vi "Turn to angle.vi"(8 "Start Time":u32, 9 "Range of accuracy":sgl, 10 "desired angle":sgl) -> (1 "In Range?":bool, 2 "coerced(x)":dbl)   [LabVIEW 2020]
doc: "turn to angle calculation in degrees"
uses:
  Robot Global Data.vi
panel:
  out "Degrees per second":dbl
  out "Diffrence":dbl
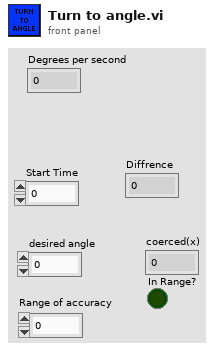
[diagram p1: front panel]
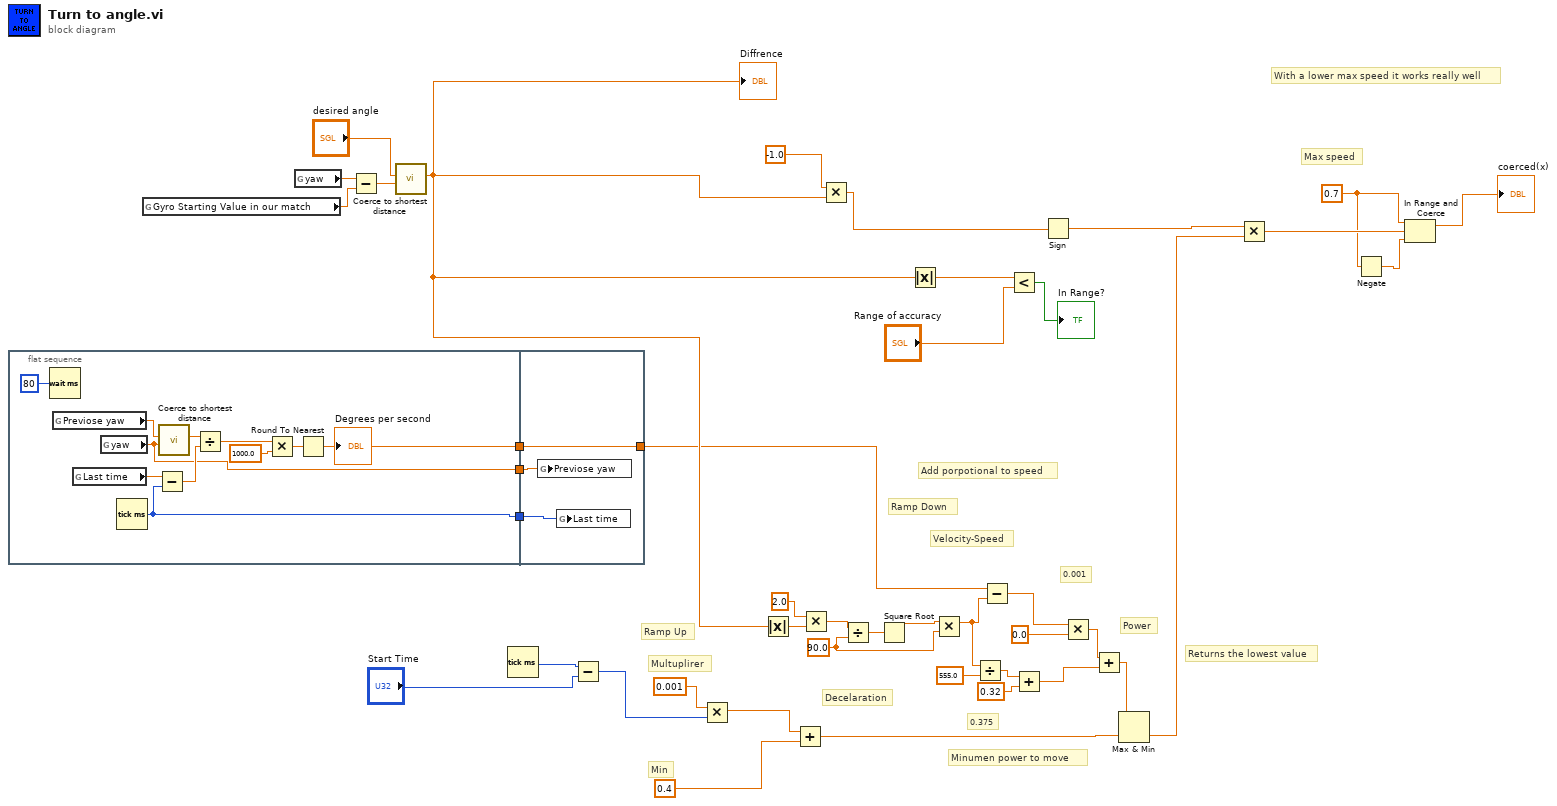
[diagram p0: block diagram]
diagram:
  w16 = 90.0 ("x")
  w33 = 0.7 ("t")
  # "0.375"
  # "0.001"
  # "Power"
  # "Minumen power to move"
  # "Add porpotional to speed"
  # "Ramp Down"
  # "Velocity-Speed"
  # "Decelaration"
  # "With a lower max speed it works really well"
  # "Multuplirer"
  # "Min"
  # "Ramp Up"
  # "Returns the lowest value"
  # "Max speed"
  n1 = flat-sequence {
    tunnel: [w51] -> w23
    tunnel: [w45] -> w22
    tunnel: [w43] -> w10
    tunnel: w23 -> [w56]
    tunnel: w22 -> [w55]
    tunnel: [w54] -> w11
    tunnel: w10 -> [w54]
    frame #0 {
      n2 = Wait (ms)(milliseconds to wait=u32 80) -> ()  [unwired: 1 out]
      n3 = global read "Robot Global Data.vi" "Previose yaw"() -> (w46:dbl)
      n4 = global read "Robot Global Data.vi" "Last time"() -> (w53:dbl)
      n5 = global read "Robot Global Data.vi" "yaw"() -> (w45:dbl)
      n6 = Tick Count (ms)() -> (millisecond timer value=w51:u32)
      n7 = Subtract(x=w53, y=w51) -> (x-y=w52:dbl)
      n8 = call "Coerce to shortest distance.vi"("Angle 2"=w45, "Angle 1"=w46) -> ("Shortest distance"=w44:dbl)  [unwired: 9 in]
      n9 = Divide(x=w44, y=w52) -> (x/y=w50:dbl)
      n10 = Multiply(x=w50, y=1000.0) -> (x*y=w47:dbl)
      n11 = Round To Nearest(number=w47) -> (nearest integer value=w43:dbl)
      "Degrees per second" <- w43
    }
    frame #1 {
      n12 = global write "Robot Global Data.vi" "Previose yaw"(w55) -> ()
      n13 = global write "Robot Global Data.vi" "Last time"(w56) -> ()
    }
  }
  n14 = global read "Robot Global Data.vi" "Gyro Starting Value in our match"() -> (w21:dbl)
  n15 = global read "Robot Global Data.vi" "yaw"() -> (w28:dbl)
  n16 = Subtract(x=w28, y=w21) -> (x-y=w13:dbl)
  n17 = call "Coerce to shortest distance.vi"("Angle 2"=w13, "Angle 1"="desired angle") -> ("Shortest distance"=w12:dbl)  [unwired: 9 in]
  "Diffrence" <- w12
  n18 = Tick Count (ms)() -> (millisecond timer value=w37:u32)
  n19 = Subtract(x=w37, y="Start Time") -> (x-y=w36:u32)
  n20 = Multiply(x=0.001 ("y"), y=w36) -> (x*y=w39:dbl)
  n21 = Absolute Value(x=w12) -> (abs(x)=w15:dbl)
  n22 = Add(x=w39, y=0.4) -> (x+y=w31:dbl)
  n23 = Multiply(x=2.0, y=w15) -> (x*y=w18:dbl)
  n24 = Multiply(x=-1.0, y=w12) -> (x*y=w27:dbl)
  n25 = Divide(x=w18, y=w16) -> (x/y=w19:dbl)
  n26 = Square Root(x=w19) -> (sqrt(x)=w17:dbl)
  n27 = Absolute Value(x=w12) -> (abs(x)=w26:dbl)
  n28 = Multiply(x=w17, y=w16) -> (x*y=w6:dbl)
  n29 = Divide(x=w6, y=555.0) -> (x/y=w8:dbl)
  n30 = Subtract(x=w11, y=w6) -> (x-y=w5:dbl)
  n31 = Less?(x=w26, y="Range of accuracy") -> (x < y?=→"In Range?":bool)
  n32 = Add(x=w8, y=0.32) -> (x+y=w2:dbl)
  n33 = Sign(1:w27) -> (0:w38:dbl)
  n34 = Multiply(x=w5, y=0.0) -> (x*y=w1:dbl)
  n35 = Add(x=w1, y=w2) -> (x+y=w3:dbl)
  n36 = Max & Min(x=w3, y=w31) -> (min(x,y)=w29:dbl)  [unwired: 1 out]
  n37 = Multiply(x=w38, y=w29) -> (x*y=w34:dbl)
  n38 = Negate(x=w33) -> (-x=w32:dbl)
  n39 = In Range and Coerce(upper limit=w33, x=w34, lower limit=w32) -> (coerced(x)=→"coerced(x)":dbl)  [unwired: 1 out]
